vi "Hardware-DiffIO.vi"(8 "error in (no error)":errorcluster, 11 "DCM-DSI in":refnum<class "DCM-DSI.lvclass">) -> (0 "error out":errorcluster, 3 "DCM-DSI out":refnum<class "DCM-DSI.lvclass">)   [LabVIEW 2016, in "DSI-RT.lvlib"]
uses:
  DSI-RT.lvlib
  Classes/DCM-DSI/DCM-DSI.lvclass
  Classes/DCM-DSI/Read DCM Ref.vi
  Classes/DCM-DSI/Read DiffIO Setup.vi
  Classes/DCM-DSI/Write DiffIO State.vi
  Classes/DCM-DSI/Write DiffIO Setup.vi
  Classes/DCM-DSI/Write DiffIO Results.vi
  <vilib>/Powertrain Controls/Device Drivers/DCM/Rev0/RT/DCM - RT.lvclass
  <vilib>/Powertrain Controls/Device Drivers/DCM/Diff IO/RT/DCM - RT - Diff IO.lvlib
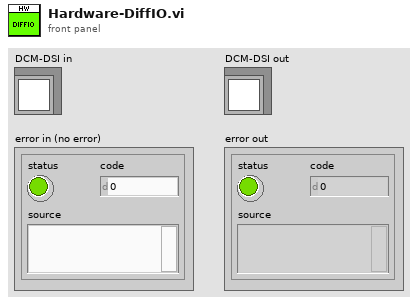
[diagram p1: front panel]
types:
  T1 = typedef "DCM - RT - Diff IO.lvlib/Setup.ctl" = cluster{"Mode":T2, "Capture Start [DBTDC]":sgl, "Capture End [DBTDC]":sgl, "Invert":bool, "Frequency [Hz]":sgl, "Duty Cycle [%]":sgl, "TDC Offset [CAD]":sgl, "Window Start [DBTDC]":sgl, "Window End [DBTDC]":sgl, "Angles":T3[], "Skip Fire":bool, "Skip Fire Index":u8}
  T2 = typedef "DCM - FPGA - Diff IO.lvlib/Mode.ctl" = enum8{"Off", "Input", "Pulse Width Modulation", "Engine Position Tracking", "Serial Out 1", "Serial Out 2", "EPTx Sync"}
  T3 = typedef "DCM - RT - Diff IO.lvlib/Angle Control.ctl" = cluster{"Enable":bool, "Location [DBTDC]":sgl, "Duration [s]":sgl}
  T4 = typedef "DCM - RT - Diff IO.lvlib/Results.ctl" = cluster{"Capture [DBTDC]":sgl, "Capture Error":bool, "Frequency [Hz]":sgl, "Duty Cycle [%]":sgl, "PWM Stopped":bool}
  T5 = typedef "DCM - FPGA - Tools.lvlib/8 Channels.ctl" = cluster{"1":bool, "2":bool, "3":bool, "4":bool, "5":bool, "6":bool, "7":bool, "8":bool}
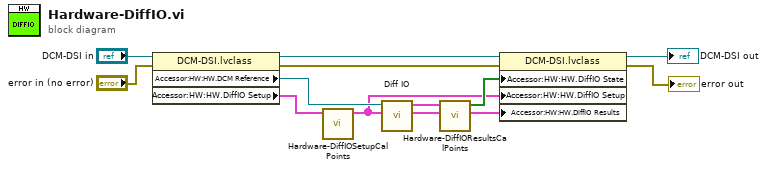
[diagram p0: block diagram]
diagram:
  n1 = property class="DCM-DSI.lvclass"(reference="DCM-DSI in", error in="error in (no error)") -> (reference out=w3:refnum<class "DCM-DSI.lvclass">, error out=w5:errorcluster, "Accessor:HW:HW.DCM Reference"=w4:refnum<class "DCM - RT.lvclass">, "Accessor:HW:HW.DiffIO Setup"=w7:T1[])
  n2 = call "Hardware-DiffIOSetupCalPoints.vi"("Diff I/O Setup"=w7) -> ("Diff I/O Setup"=w1:T1[])  [unwired: 10 in]
  n3 = call <vilib>:"Diff IO.vi"("Diff IO Setup"=w1, "DCM Reference"=w4) -> ("Diff IO Results"=w2:T4[], "Diff IO In"=w8:T5)  [unwired: 8 in]
  n4 = call "Hardware-DiffIOResultsCalPoints.vi"("Diff IO Results"=w2, "DIFF I/O State"=w8) -> ("DiffIO State"=w6:bool[])  [unwired: 9 in]
  n5 = property class="DCM-DSI.lvclass"(reference=w3, error in=w5, "Accessor:HW:HW.DiffIO State"=w6, "Accessor:HW:HW.DiffIO Setup"=w1, "Accessor:HW:HW.DiffIO Results"=w2) -> (reference out=→"DCM-DSI out":refnum<class "DCM-DSI.lvclass">, error out=→"error out":errorcluster)
